vi "SV TDMS Write Spectrum Info.vi"(0 "tdms file":refnum<k34>, 1 "spectrum component":T7=32 items=["Magnitude"=32, "Phase"=33, "Real"=34, "Imaginary"=35, "Coherence"=36, "Unknown"=99], 2 "spectrum info":T8 {"x-axis units" items=["Time (s)"=0, "Frequency-CB (Hz)"=1, "Frequency-CPB (Hz)"=1248, "Frequency-Arbitrary (Hz)"=2357, "Quefrency (s)"=2, "Revolutions (rev)"=3, "Order"=4, "Speed (RPM)"=11, "Speed (rad/s)"=21, "Index"=65535]; "weighting filter" items=["Linear", "A-weighting", "B-weighting", "C-weighting", "ITU-R 468-4", "Dolby", "CCITT", "C-message", "Wb", "Wc", "Wd", "We", "Wf", "Wh", "Wj", "Wk", "Wm", "AES17 20 kHz lowpass", "AES17 40 kHz lowpass", "AES17 20 kHz highpass", "AES17 40 kHz highpass"]; "dB reference [EU]" format="%.2f"; "engineering units" items=["custom..."=0, "V"=1, "A"=21, "C"=30, "pC"=31, "s"=32, "-"=29, "Pa"=2, "N"=20, "g"=3, "m/s^2"=4, "m/s"=5, "m"=6, "mm/s"=12, "mm"=13, "micron/s"=14, "micron"=15, "in/s^2"=7, "in/s"=8, "in"=9, "mil/s"=10, "mil"=11, "rad/s^2"=16, "rad/s"=17, "rad"=18, "deg/s^2"=26, "deg/s"=27, "deg"=28, "RPM"=22, "cycle/s^2"=23, "Hz"=24, "cycle"=25, "strain"=19]; "spectral info"."window" items=["None "=0, "Hanning"=1, "Hamming"=2, "Blackman-Harris"=3, "Exact Blackman"=4, "Blackman"=5, "Flat Top"=6, "4 Term B-Harris "=7, "7 Term B-Harris"=8, "Low Sidelobe"=9, "Force - Exponential"=10, "Gaussian"=62]}, 3 "LabVIEW datatype":T1=3 items=["String: abc"=7, "Boolean: True or False"=8, "Scalar: y"=0, "Array: Y"=1, "Waveform: t0, dt, Y, variant"=2, "Cluster: x0, dx, Y"=3, "Cluster: X, Y"=4, "Waterfall"=5, "Colormap"=6], 5 "group name in":string, 7 "channel name in":string, 11 "error in":errorcluster) -> (4 "tdms file out":refnum<k34>, 6 "group name out":string, 8 "channel name out":string, 13 "function info":T6 {"function type" items=["Signal"=0, "Speed"=3, "Ratio"=6, "Count"=7, "-"=9, "Level"=10, "-"=19, "Octave Spectrum"=20, "-"=29, "FFT Auto Spectrum"=30, "FFT Cross Spectrum"=40, "Frequency Response"=50, "-"=59, "Event"=90]; "function subtype" items=["Unscaled binary"=0, "Scaled voltage"=1, "Scaled engineering units"=2, "-"=10, "Value"=19, "DC"=11, "AC"=12, "RMS^2"=13, "RMS"=14, "Peak"=15, "Peak to peak"=16, "-"=20, "1/1 octave"=21, "1/3 octave"=22, "1/6 octave"=23, "1/12 octave"=24, "1/24 octave"=25, "-"=30, "Density"=31, "Magnitude"=32, "Phase"=33, "Real"=34, "Imaginary"=35, "Complex"=345, "Coherence"=36, "-"=90, "Unknown"=99]; "X-domain" items=["Time (s)"=0, "Frequency-CB (Hz)"=1, "Frequency-CPB (Hz)"=1248, "Frequency-Arbitrary (Hz)"=2357, "Quefrency (s)"=2, "Revolutions (rev)"=3, "Order"=4, "Speed (RPM)"=11, "Speed (rad/s)"=21, "Index"=65535]}, 14 "unit info":T2, 15 "error out":errorcluster)   [LabVIEW 2017]
uses:
  <vilib>/addons/_NISVFA/_Shared subVIs/Controls/svc_Spectrum Info.ctl
  <vilib>/addons/_NISVFA/_Shared subVIs/Controls/svc_X-Axis Units.ctl
  <vilib>/addons/_NISVFA/_Shared subVIs/Controls/svc_Spectrum Type.ctl
  <vilib>/addons/_NISVFA/_Shared subVIs/Controls/svc_Engineering Units Text Ring.ctl
  <vilib>/addons/_NISVFA/_Shared subVIs/Controls/svc_Weighting Filter Text Ring.ctl
  <vilib>/addons/_NISVFA/_Shared subVIs/Controls/svc_Complimentary Spectrum Units.ctl
  <vilib>/addons/_NISVFA/_Shared subVIs/Controls/NI Spectrum Component.ctl
  <vilib>/addons/_NISVFA/_Shared subVIs/Controls/NI Function Type.ctl
  <vilib>/addons/_NISVFA/_Shared subVIs/Controls/NI Function SubType.ctl
  <vilib>/addons/_NISVFA/_Shared subVIs/Controls/LV Datatypes.ctl
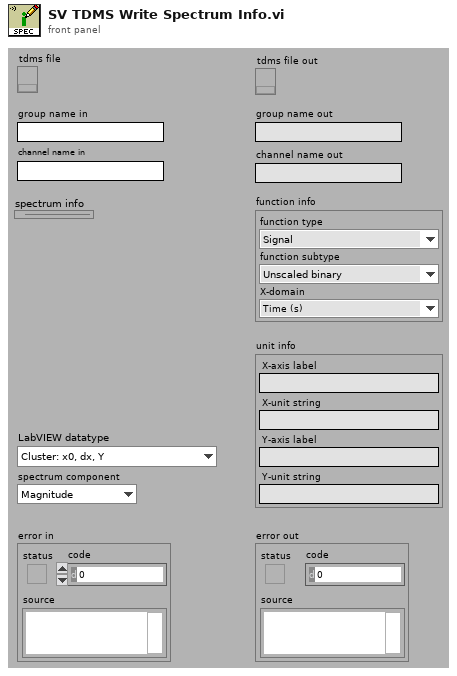
[diagram p1: front panel]
types:
  T1 = typedef "LV Datatypes.ctl" = i32
  T2 = cluster{"X-axis label":string, "X-unit string":string, "Y-axis label":string, "Y-unit string":string}
  T3 = typedef "NI Function Type.ctl" = u16
  T4 = typedef "NI Function SubType.ctl" = u16
  T5 = typedef "svc_X-Axis Units.ctl" = u16
  T6 = cluster{"function type":T3, "function subtype":T4, "X-domain":T5}
  T7 = typedef "NI Spectrum Component.ctl" = u16
  T8 = typedef "svc_Spectrum Info.ctl" = cluster{"channel name":string, "description":string, "x-axis units":T5, "spectral info":cluster{"spectrum type":T9, "linear/dB":enum16{"linear", "dB"}, "window":u16, "window size":i32, "FFT size":i32}, "engineering units":T10, "custom label":string, "dB reference [EU]":dbl, "peak units":enum16{"rms", "peak", "peak-peak"}, "weighting filter":T11, "spectral density?":bool, "unit label":string, "spectrum skewed?":bool, "complimentary spectrum units":T12}
  T9 = typedef "svc_Spectrum Type.ctl" = enum16{"FFT Spectrum [complex]", "Amplitude [Magnitude]", "Power [Magnitude^2]", "Cross Spectrum [complex]", "Frequency Response [Complex]"}
  T10 = typedef "svc_Engineering Units Text Ring.ctl" = u16
  T11 = typedef "svc_Weighting Filter Text Ring.ctl" = u16
  T12 = typedef "svc_Complimentary Spectrum Units.ctl" = enum16{"none", "radians", "degrees", "cycles", "imaginary"}
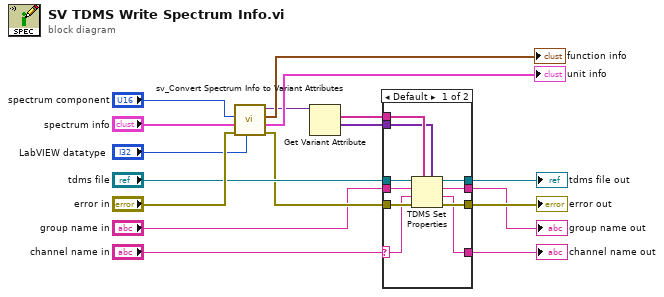
[diagram p0: block diagram]
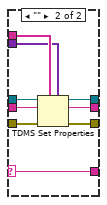
[diagram p2: hidden frame]
diagram:
  n1 = call <vilib>:"sv_Convert Spectrum Info to Variant Attributes.vi"("LabVIEW datatype"="LabVIEW datatype", "error in"="error in", "spectrum info"="spectrum info", "spectrum component"="spectrum component") -> ("error out"=w12:errorcluster, "unit info"=→"unit info":T2, "function info"=→"function info":T6, "attributes out"=w3:variant)  [unwired: 4 in]
  n2 = Get Variant Attribute(Variant=w3) -> (names=w1:string[], values=w2:variant[])  [unwired: 3 in, 2 out]
  n3 = case shown="Default" "channel name in" {
    selector: "channel name in" -> [w18 w28]
    tunnel: "tdms file" -> [w27 w36]
    tunnel: w12 -> [w26 w35]
    tunnel: [w25 w34] -> w11
    tunnel: "group name in" -> [w24 w33]
    tunnel: w1 -> [w23 w32]
    tunnel: w2 -> [w22 w31]
    tunnel: [w21 w30] -> w9
    tunnel: [w20 w29] -> w8
    tunnel: [w19 w28] -> w7
    frame Default {
      n4 = TDMS Set Properties(5:w22, 7:w23, 8:w26, 9:w18, 10:w24, 11:w27) -> (0:w25:errorcluster, 1:w19:string, 2:w20:string, 3:w21:refnum<k34>)
    }
    frame "" {
      n5 = TDMS Set Properties(5:w31, 7:w32, 8:w35, 10:w33, 11:w36) -> (0:w34:errorcluster, 2:w29:string, 3:w30:refnum<k34>)  [unwired: 1 in, 1 out]
    }
  }
  "tdms file out" <- w9
  "group name out" <- w8
  "channel name out" <- w7
  "error out" <- w11
